vi "Generate JSON Schema VCluster.vi"(6 "strict?":bool, 8 "error in (no error)":errorcluster, 11 "type":variant) -> (0 "error out":errorcluster, 3 "json schema cluster":variant)   [LabVIEW 2023]
uses:
  <vilib>/Utility/Data Type/NI_Data Type.lvlib
  <userlib>/_OpenG.lib/lvdata/lvdata.llb/openg_variant.lvlib
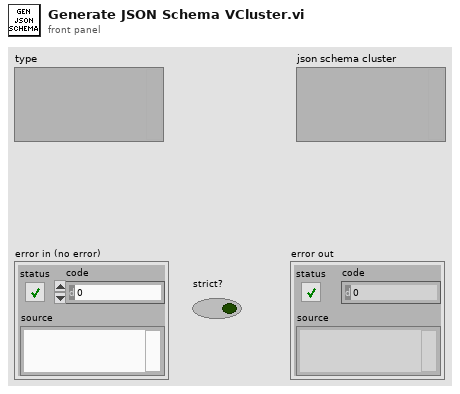
[diagram p1: front panel]
types:
  T1 = typedef "NI_Data Type.lvlib/Data Type.ctl" = enum8{"Invalid Type", "Void", "I8", "I16", "I32", "I64", "U8", "U16", "U32", "U64", "Single Float", "Double Float", "Extended Float", "Single Complex", "Double Complex", "Extended Complex", "Enum U8", "Enum U16", "Enum U32", "Enum U64", "Single Float With Unit", "Double Float With Unit", "Extended Float With Unit", "Single Complex with Unit", "Double Complex with Unit", "Extended Complex with Unit", "Boolean", "String", "Path", "Picture", "Tag", "Array", "Cluster", "Variant", "LV Variant", "Waveform", "Timestamp", "Digital Waveform", "Digital Data", "ExpressData", "Refnum", "External Data", "VI", "Poly VI", "LabVIEW Class Instance", "Fixed Point", "Set Collection", "Map Collection"}
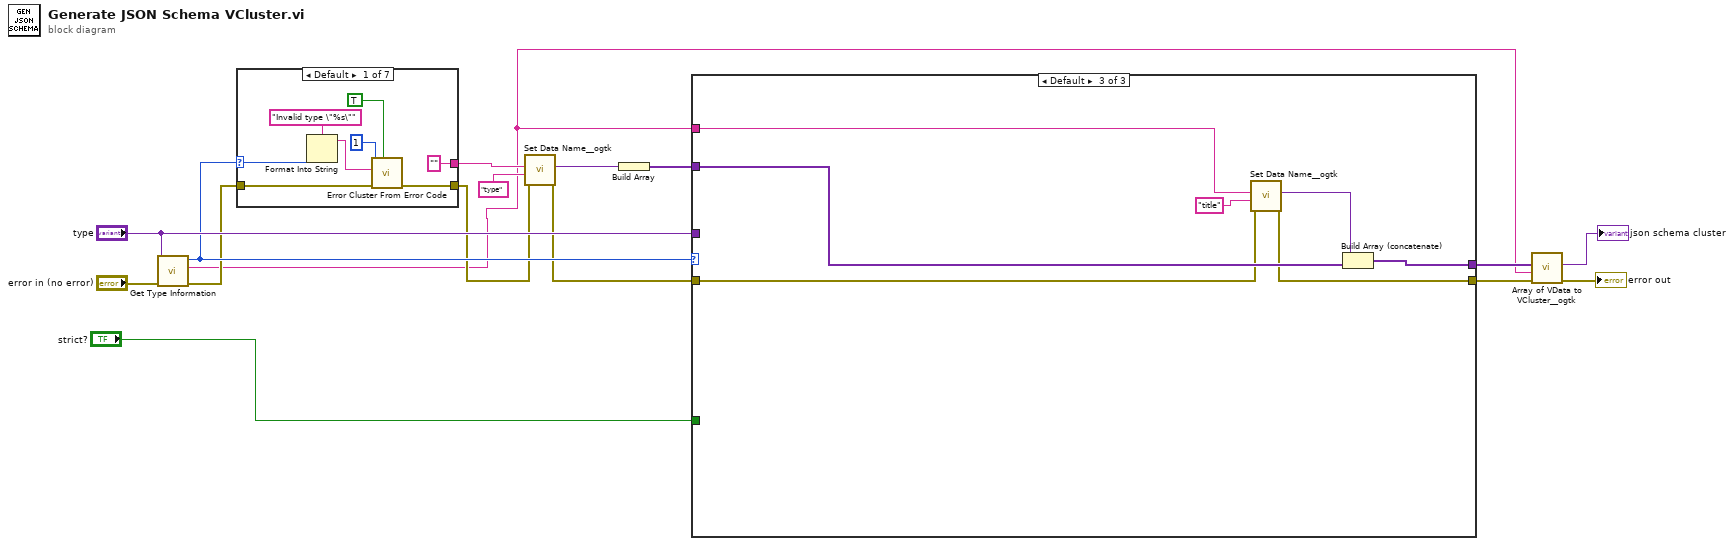
[diagram p0: block diagram]
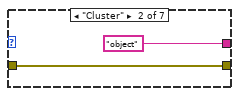
[diagram p2: hidden frame]
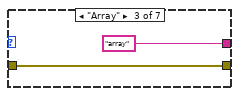
[diagram p3: hidden frame]
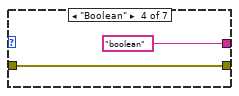
[diagram p4: hidden frame]
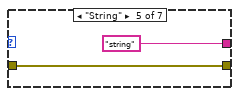
[diagram p5: hidden frame]
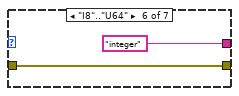
[diagram p6: hidden frame]
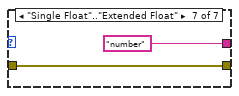
[diagram p7: hidden frame]
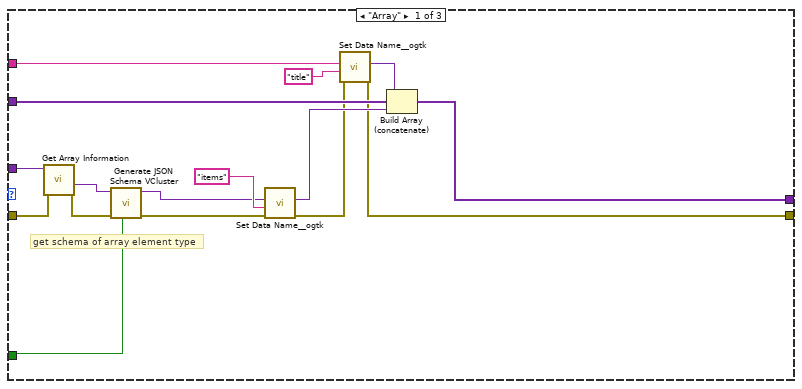
[diagram p8: hidden frame]
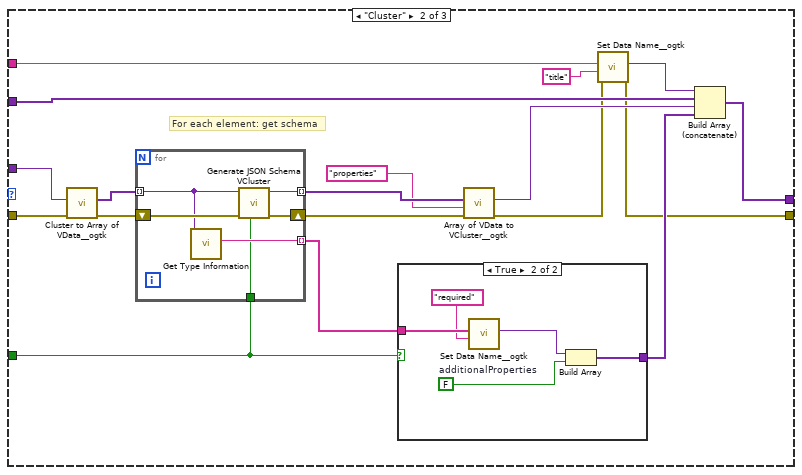
[diagram p9: hidden frame]
diagram:
  n1 = call <vilib>:"Get Type Information.vi"("error in (no error)"="error in (no error)", "variant"="type") -> ("error out"=w7:errorcluster, "name"=w2:string, "type"=w8:T1)  [unwired: 5 in, 2 out]
  n2 = case shown="Default" w8 {
    selector: w8 -> [w20 _ _ _ _ _ _]
    tunnel: ["" ("name") "object" ("name") "array" ("name") "boolean" ("name") "string" ("name") "integer" ("name") "number" ("name")] -> w14
    tunnel: [w22 w25 w27 w29 w31 w33 w35] -> w5
    tunnel: w7 -> [w24 w25 w27 w29 w31 w33 w35]
    frame Default {
      n3 = Format Into String(format string="Invalid type \"%s\"", w20) -> (resulting string=w18:string)  [unwired: 2 in, 1 out]
      n4 = call <vilib>:"Error Cluster From Error Code.vi"("show call chain? (False)"=TRUE, "error in (no error)"=w24, "error message (\"\")"=w18, "error code (0)"=1) -> ("error out"=w22:errorcluster)  [unwired: 5 in]
    }
    frame "Cluster" {
    }
    frame "Array" {
    }
    frame "Boolean" {
    }
    frame "String" {
    }
    frame "I8".."U64" {
    }
    frame "Single Float".."Extended Float" {
    }
  }
  n5 = call <userlib>:"Set Data Name__ogtk.vi"("error in (no error)"=w5, "Data Name"="type" ("name"), "Data"=w14) -> ("error out"=w1:errorcluster, "Renamed Data"=w12:variant)  [unwired: 7 in]
  n6 = Build Array(w12) -> (w11:variant[])
  n7 = case shown="Default" w8 {
    tunnel: [w46 w64 w85] -> w10
    tunnel: "type" -> [w52 w70 _]
    tunnel: w11 -> [w47 w68 w88]
    tunnel: w1 -> [w45 w63 w82]
    tunnel: [w37 w53 w83] -> w4
    tunnel: "strict?" -> [w42 w58 _]
    tunnel: w2 -> [w41 w56 w86]
    frame "Array" {
      # "get schema of array element type"
      n8 = call <vilib>:"Get Array Information.vi"("error in (no error)"=w45, "variant"=w52) -> ("error out"=w44:errorcluster, "array element data type"=w51:variant)  [unwired: 6 in, 2 out]
      n9 = call "Generate JSON Schema VCluster.vi"("strict?"=w42, "error in (no error)"=w44, "type"=w51) -> ("error out"=w43:errorcluster, "json schema cluster"=w49:variant)  [unwired: 7 in]
      n10 = call <userlib>:"Set Data Name__ogtk.vi"("error in (no error)"=w43, "Data Name"="items" ("name"), "Data"=w49) -> ("error out"=w38:errorcluster, "Renamed Data"=w48:variant)  [unwired: 7 in]
      n11 = call <userlib>:"Set Data Name__ogtk.vi"("error in (no error)"=w38, "Data Name"="title" ("name"), "Data"=w41) -> ("error out"=w37:errorcluster, "Renamed Data"=w39:variant)  [unwired: 7 in]
      n12 = Build Array (concatenate)(w39, w47, w48) -> (w46:variant[])
    }
    frame "Cluster" {
      # "For each element: get schema"
      n13 = call <userlib>:"Cluster to Array of VData__ogtk.vi"("error in (no error)"=w63, "Cluster"=w70) -> ("error out"=w62:errorcluster, "Array of VData"=w69:variant[])  [unwired: 8 in]
      n14 = for {
        tunnel: w69 -> [w78] mode=indexing
        tunnel: [w81] -> w67 mode=indexing
        shift-right: [w79] -> w61
        shift-left: w62 -> [w80]
        tunnel: [w77] -> w60 mode=indexing
        tunnel: w58 -> [w76]
        n15 = call <vilib>:"Get Type Information.vi"("variant"=w78) -> ("name"=w77:string)  [unwired: 6 in, 4 out]
        n16 = call "Generate JSON Schema VCluster.vi"("strict?"=w76, "error in (no error)"=w80, "type"=w78) -> ("error out"=w79:errorcluster, "json schema cluster"=w81:variant)  [unwired: 7 in]
      }
      n17 = case shown="True" w58 {
        tunnel: w60 -> [_ w75]
        tunnel: [_ w71] -> w59
        frame False {
        }
        frame True {
          w72 = FALSE  # additionalProperties
          n18 = call <userlib>:"Set Data Name__ogtk.vi"("Data Name"="required" ("name"), "Data"=w75) -> ("Renamed Data"=w73:variant)  [unwired: 8 in, 1 out]
          n19 = Build Array(w73, w72) -> (w71:variant[])
        }
      }
      n20 = call <userlib>:"Array of VData to VCluster__ogtk.vi"("error in (no error)"=w61, "Cluster Name"="properties" ("name"), "Array"=w67) -> ("error out"=w54:errorcluster, "VCluster"=w65:variant)  [unwired: 7 in]
      n21 = call <userlib>:"Set Data Name__ogtk.vi"("error in (no error)"=w54, "Data Name"="title" ("name"), "Data"=w56) -> ("error out"=w53:errorcluster, "Renamed Data"=w55:variant)  [unwired: 7 in]
      n22 = Build Array (concatenate)(w55, w68, w65, w59) -> (w64:variant[])
    }
    frame Default {
      n23 = call <userlib>:"Set Data Name__ogtk.vi"("error in (no error)"=w82, "Data Name"="title" ("name"), "Data"=w86) -> ("error out"=w83:errorcluster, "Renamed Data"=w84:variant)  [unwired: 7 in]
      n24 = Build Array (concatenate)(w84, w88) -> (w85:variant[])
    }
  }
  n25 = call <userlib>:"Array of VData to VCluster__ogtk.vi"("error in (no error)"=w4, "Cluster Name"=w2, "Array"=w10) -> ("error out"=→"error out":errorcluster, "VCluster"=→"json schema cluster":variant)  [unwired: 7 in]
